vi "test_Compare Test Object Accessors.vi"() -> ()   [LabVIEW 2015]
uses:
  Test Object/Test Object.lvclass
  Test Object/Test Object.lvclass/Test Object.ctl
  Test Object/Read Variant (sta prop).vi
  Test Object/Write Variant (sta prop).vi
panel:
  out "Average test duration [ms]":dbl[][](array[numeric]) format="%#.6p"
  # "Access Variant w/o modification"
  # "Access and modify Variant in-place"
  # "Access and reallocate Variant"
  # "Static w/o errors"
  # "Dynam w/o errors"
  # "Static prop"
  # "Dynam prop"
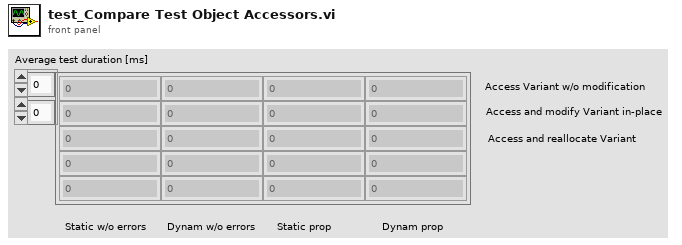
[diagram p1: front panel]
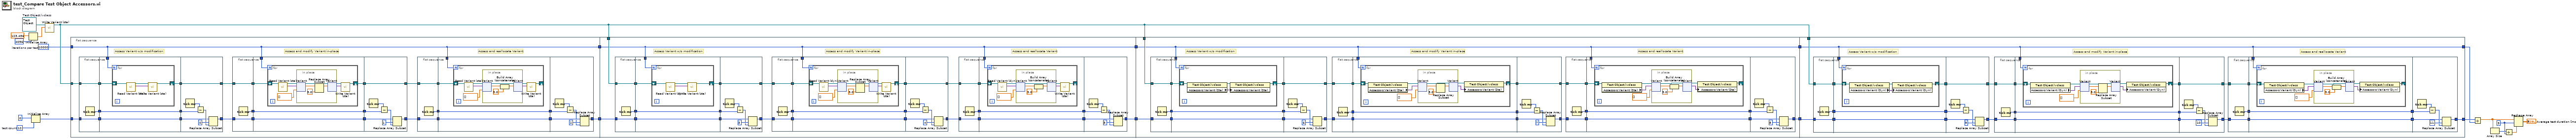
[diagram p0: block diagram]
diagram:
  w6 = 10000  # iterations per test
  w8 = 3
  w16 = 12  # test count
  w22 = refnum<class "Test Object.lvclass"> refnum  # Test Object.lvclass
  n1 = Initialize Array(123.456, 4096) -> (w19:dbl[])
  n2 = Initialize Array(u32 0, w16) -> (w15:u32[])
  n3 = call "Write Variant (sta).vi"("Variant"=w19, "Test Object in"=w22) -> ("Test Object out"=w18:refnum<class "Test Object.lvclass">)  [unwired: 9 in]
  n4 = flat-sequence {
    tunnel: w18 -> [w34]
    tunnel: w15 -> [w33]
    tunnel: [w24] -> w14
    tunnel: w6 -> [w23]
    tunnel: [w23] -> w5
    tunnel: w18 -> [w116]
    tunnel: w14 -> [w115]
    tunnel: [w114] -> w13
    tunnel: w5 -> [w113]
    tunnel: [w113] -> w4
    tunnel: w18 -> [w214]
    tunnel: w13 -> [w211]
    tunnel: [w204] -> w12
    tunnel: w4 -> [w203]
    tunnel: [w203] -> w3
    tunnel: w18 -> [w296]
    tunnel: w12 -> [w295]
    tunnel: [w294] -> w10
    tunnel: w3 -> [w293]
    tunnel: [w293] -> w1
    frame #0 {
      # "Access and reallocate Variant"
      # "Access and modify Variant in-place"
      # "Access Variant w/o modification"
      n5 = flat-sequence {
        tunnel: w34 -> [w96]
        tunnel: [w96] -> w47
        tunnel: [w95] -> w46
        tunnel: w33 -> [w94]
        tunnel: [w94] -> w32
        tunnel: w47 -> [w101]
        tunnel: w46 -> [w99]
        tunnel: [w100] -> w45
        tunnel: [w99] -> w44
        tunnel: w32 -> [w98]
        tunnel: [w98] -> w31
        tunnel: w23 -> [w97]
        tunnel: [w112] -> w35
        tunnel: w45 -> [w112]
        tunnel: w44 -> [w111]
        tunnel: w31 -> [w107]
        tunnel: [w106] -> w29
        frame #0 {
          n6 = Tick Count (ms)() -> (millisecond timer value=w95:u32)
        }
        frame #1 {
          n7 = for {
            N: w97 -> [_]
            shift-right: [w103] -> w100
            shift-left: w101 -> [w105]
            n8 = call "Read Variant (sta).vi"("Test Object in"=w105) -> ("Variant"=w102:variant, "Test Object out"=w104:refnum<class "Test Object.lvclass">)  [unwired: 9 in]
            n9 = call "Write Variant (sta).vi"("Variant"=w102, "Test Object in"=w104) -> ("Test Object out"=w103:refnum<class "Test Object.lvclass">)  [unwired: 9 in]
          }
        }
        frame #2 {
          n10 = Tick Count (ms)() -> (millisecond timer value=w110:u32)
          n11 = Subtract(x=w110, y=w111) -> (x-y=w108:u32)
          n12 = Replace Array Subset(array=w107, new element=w108, index=0) -> (w106:u32[])
        }
      }
      n13 = flat-sequence {
        tunnel: w35 -> [w72]
        tunnel: [w72] -> w43
        tunnel: [w71] -> w42
        tunnel: [w70] -> w30
        tunnel: w29 -> [w70]
        tunnel: w43 -> [w77]
        tunnel: w42 -> [w75]
        tunnel: [w76] -> w41
        tunnel: [w75] -> w40
        tunnel: w30 -> [w74]
        tunnel: [w74] -> w28
        tunnel: w23 -> [w73]
        tunnel: [w93] -> w36
        tunnel: w41 -> [w93]
        tunnel: w40 -> [w92]
        tunnel: w28 -> [w88]
        tunnel: [w87] -> w26
        frame #0 {
          n14 = Tick Count (ms)() -> (millisecond timer value=w71:u32)
        }
        frame #1 {
          n15 = for {
            N: w73 -> [_]
            shift-right: [w81] -> w76
            shift-left: w77 -> [w83]
            n16 = call "Read Variant (sta).vi"("Test Object in"=w83) -> ("Variant"=w80:variant, "Test Object out"=w82:refnum<class "Test Object.lvclass">)  [unwired: 9 in]
            n17 = in-place {
              n18 = in-place-variant #1(w80, dbl[] []) -> (w86:dbl[])  [unwired: 1 out]
              n19 = Replace Array Subset(array=w86, new element=5.0) -> (w85:dbl[])  [unwired: 1 in]
              n20 = in-place-variant #1(w85) -> (w79:variant)  [unwired: 1 out]
            }
            n21 = call "Write Variant (sta).vi"("Variant"=w79, "Test Object in"=w82) -> ("Test Object out"=w81:refnum<class "Test Object.lvclass">)  [unwired: 9 in]
          }
        }
        frame #2 {
          n22 = Tick Count (ms)() -> (millisecond timer value=w91:u32)
          n23 = Subtract(x=w91, y=w92) -> (x-y=w89:u32)
          n24 = Replace Array Subset(array=w88, new element=w89, index=1) -> (w87:u32[])
        }
      }
      n25 = flat-sequence {
        tunnel: w36 -> [w50]
        tunnel: [w50] -> w39
        tunnel: [w49] -> w38
        tunnel: [w48] -> w27
        tunnel: w26 -> [w48]
        tunnel: w39 -> [w54]
        tunnel: w38 -> [w53]
        tunnel: [w53] -> w37
        tunnel: w27 -> [w52]
        tunnel: [w52] -> w25
        tunnel: w23 -> [w51]
        tunnel: w37 -> [w69]
        tunnel: w25 -> [w66]
        tunnel: [w64] -> w24
        frame #0 {
          n26 = Tick Count (ms)() -> (millisecond timer value=w49:u32)
        }
        frame #1 {
          n27 = for {
            N: w51 -> [_]
            shift-right: [w58] -> _
            shift-left: w54 -> [w60]
            n28 = call "Read Variant (sta).vi"("Test Object in"=w60) -> ("Variant"=w57:variant, "Test Object out"=w59:refnum<class "Test Object.lvclass">)  [unwired: 9 in]
            n29 = in-place {
              n30 = in-place-variant #2(w57, dbl[] []) -> (w63:dbl[])  [unwired: 1 out]
              n31 = Build Array (concatenate)(w63, 5.0) -> (w62:dbl[])
              n32 = in-place-variant #2(w62) -> (w56:variant)  [unwired: 1 out]
            }
            n33 = call "Write Variant (sta).vi"("Variant"=w56, "Test Object in"=w59) -> ("Test Object out"=w58:refnum<class "Test Object.lvclass">)  [unwired: 9 in]
          }
        }
        frame #2 {
          n34 = Tick Count (ms)() -> (millisecond timer value=w68:u32)
          n35 = Subtract(x=w68, y=w69) -> (x-y=w65:u32)
          n36 = Replace Array Subset(array=w66, new element=w65, index=2) -> (w64:u32[])
        }
      }
    }
    frame #1 {
      # "Access and reallocate Variant"
      # "Access and modify Variant in-place"
      # "Access Variant w/o modification"
      n37 = flat-sequence {
        tunnel: w116 -> [w186]
        tunnel: [w186] -> w137
        tunnel: [w185] -> w136
        tunnel: w115 -> [w184]
        tunnel: [w184] -> w135
        tunnel: w137 -> [w191]
        tunnel: w136 -> [w189]
        tunnel: [w190] -> w134
        tunnel: [w189] -> w133
        tunnel: w135 -> [w188]
        tunnel: [w188] -> w132
        tunnel: w113 -> [w187]
        tunnel: [w202] -> w119
        tunnel: w134 -> [w202]
        tunnel: w133 -> [w201]
        tunnel: w132 -> [w197]
        tunnel: [w196] -> w118
        frame #0 {
          n38 = Tick Count (ms)() -> (millisecond timer value=w185:u32)
        }
        frame #1 {
          n39 = for {
            N: w187 -> [_]
            shift-right: [w193] -> w190
            shift-left: w191 -> [w195]
            n40 = call-dynamic "Read Variant (dyn).vi"("Test Object in"=w195) -> ("Variant"=w192:variant, "Test Object out"=w194:refnum<class "Test Object.lvclass">)  [unwired: 9 in]
            n41 = call "Write Variant (sta).vi"("Variant"=w192, "Test Object in"=w194) -> ("Test Object out"=w193:refnum<class "Test Object.lvclass">)  [unwired: 9 in]
          }
        }
        frame #2 {
          n42 = Tick Count (ms)() -> (millisecond timer value=w200:u32)
          n43 = Subtract(x=w200, y=w201) -> (x-y=w198:u32)
          n44 = Replace Array Subset(array=w197, new element=w198, index=3) -> (w196:u32[])
        }
      }
      n45 = flat-sequence {
        tunnel: w119 -> [w162]
        tunnel: [w162] -> w131
        tunnel: [w161] -> w130
        tunnel: [w160] -> w129
        tunnel: w118 -> [w160]
        tunnel: w131 -> [w167]
        tunnel: w130 -> [w165]
        tunnel: [w166] -> w128
        tunnel: [w165] -> w127
        tunnel: w129 -> [w164]
        tunnel: [w164] -> w126
        tunnel: w113 -> [w163]
        tunnel: [w183] -> w120
        tunnel: w128 -> [w183]
        tunnel: w127 -> [w182]
        tunnel: w126 -> [w178]
        tunnel: [w177] -> w117
        frame #0 {
          n46 = Tick Count (ms)() -> (millisecond timer value=w161:u32)
        }
        frame #1 {
          n47 = for {
            N: w163 -> [_]
            shift-right: [w171] -> w166
            shift-left: w167 -> [w173]
            n48 = call-dynamic "Read Variant (dyn).vi"("Test Object in"=w173) -> ("Variant"=w170:variant, "Test Object out"=w172:refnum<class "Test Object.lvclass">)  [unwired: 9 in]
            n49 = in-place {
              n50 = in-place-variant #3(w170, dbl[] []) -> (w176:dbl[])  [unwired: 1 out]
              n51 = Replace Array Subset(array=w176, new element=5.0) -> (w175:dbl[])  [unwired: 1 in]
              n52 = in-place-variant #3(w175) -> (w169:variant)  [unwired: 1 out]
            }
            n53 = call "Write Variant (sta).vi"("Variant"=w169, "Test Object in"=w172) -> ("Test Object out"=w171:refnum<class "Test Object.lvclass">)  [unwired: 9 in]
          }
        }
        frame #2 {
          n54 = Tick Count (ms)() -> (millisecond timer value=w181:u32)
          n55 = Subtract(x=w181, y=w182) -> (x-y=w179:u32)
          n56 = Replace Array Subset(array=w178, new element=w179, index=4) -> (w177:u32[])
        }
      }
      n57 = flat-sequence {
        tunnel: w120 -> [w140]
        tunnel: [w140] -> w125
        tunnel: [w139] -> w124
        tunnel: [w138] -> w123
        tunnel: w117 -> [w138]
        tunnel: w125 -> [w144]
        tunnel: w124 -> [w143]
        tunnel: [w143] -> w122
        tunnel: w123 -> [w142]
        tunnel: [w142] -> w121
        tunnel: w113 -> [w141]
        tunnel: w122 -> [w159]
        tunnel: w121 -> [w156]
        tunnel: [w154] -> w114
        frame #0 {
          n58 = Tick Count (ms)() -> (millisecond timer value=w139:u32)
        }
        frame #1 {
          n59 = for {
            N: w141 -> [_]
            shift-right: [w148] -> _
            shift-left: w144 -> [w150]
            n60 = call-dynamic "Read Variant (dyn).vi"("Test Object in"=w150) -> ("Variant"=w147:variant, "Test Object out"=w149:refnum<class "Test Object.lvclass">)  [unwired: 9 in]
            n61 = in-place {
              n62 = in-place-variant #4(w147, dbl[] []) -> (w153:dbl[])  [unwired: 1 out]
              n63 = Build Array (concatenate)(w153, 5.0) -> (w152:dbl[])
              n64 = in-place-variant #4(w152) -> (w146:variant)  [unwired: 1 out]
            }
            n65 = call "Write Variant (sta).vi"("Variant"=w146, "Test Object in"=w149) -> ("Test Object out"=w148:refnum<class "Test Object.lvclass">)  [unwired: 9 in]
          }
        }
        frame #2 {
          n66 = Tick Count (ms)() -> (millisecond timer value=w158:u32)
          n67 = Subtract(x=w158, y=w159) -> (x-y=w155:u32)
          n68 = Replace Array Subset(array=w156, new element=w155, index=5) -> (w154:u32[])
        }
      }
    }
    frame #2 {
      # "Access and reallocate Variant"
      # "Access and modify Variant in-place"
      # "Access Variant w/o modification"
      n69 = flat-sequence {
        tunnel: w214 -> [w276]
        tunnel: [w276] -> w227
        tunnel: [w275] -> w226
        tunnel: [w274] -> w212
        tunnel: w211 -> [w274]
        tunnel: w227 -> [w281]
        tunnel: w226 -> [w279]
        tunnel: [w280] -> w225
        tunnel: [w279] -> w224
        tunnel: [w278] -> w213
        tunnel: w212 -> [w278]
        tunnel: w203 -> [w277]
        tunnel: [w292] -> w216
        tunnel: w225 -> [w292]
        tunnel: w224 -> [w291]
        tunnel: w213 -> [w288]
        tunnel: [w286] -> w208
        frame #0 {
          n70 = Tick Count (ms)() -> (millisecond timer value=w275:u32)
        }
        frame #1 {
          n71 = for {
            N: w277 -> [_]
            shift-right: [w283] -> w280
            shift-left: w281 -> [w285]
            n72 = property class="Test Object.lvclass"(reference=w285) -> (reference out=w284:refnum<class "Test Object.lvclass">, "Accessors:Variant (Sta)"=w282:variant)  [unwired: 1 in, 1 out]
            n73 = property class="Test Object.lvclass"(reference=w284, "Accessors:Variant (Sta)"=w282) -> (reference out=w283:refnum<class "Test Object.lvclass">)  [unwired: 1 in, 1 out]
          }
        }
        frame #2 {
          n74 = Tick Count (ms)() -> (millisecond timer value=w290:u32)
          n75 = Subtract(x=w290, y=w291) -> (x-y=w287:u32)
          n76 = Replace Array Subset(array=w288, new element=w287, index=6) -> (w286:u32[])
        }
      }
      n77 = flat-sequence {
        tunnel: w216 -> [w252]
        tunnel: [w252] -> w223
        tunnel: [w251] -> w222
        tunnel: [w250] -> w209
        tunnel: w208 -> [w250]
        tunnel: w223 -> [w257]
        tunnel: w222 -> [w255]
        tunnel: [w256] -> w221
        tunnel: [w255] -> w220
        tunnel: [w254] -> w210
        tunnel: w209 -> [w254]
        tunnel: w203 -> [w253]
        tunnel: [w273] -> w215
        tunnel: w221 -> [w273]
        tunnel: w220 -> [w272]
        tunnel: w210 -> [w268]
        tunnel: [w267] -> w206
        frame #0 {
          n78 = Tick Count (ms)() -> (millisecond timer value=w251:u32)
        }
        frame #1 {
          n79 = for {
            N: w253 -> [_]
            shift-right: [w261] -> w256
            shift-left: w257 -> [w263]
            n80 = property class="Test Object.lvclass"(reference=w263) -> (reference out=w262:refnum<class "Test Object.lvclass">, "Accessors:Variant (Sta)"=w259:variant)  [unwired: 1 in, 1 out]
            n81 = in-place {
              n82 = in-place-variant #5(w259, dbl[] []) -> (w266:dbl[])  [unwired: 1 out]
              n83 = Replace Array Subset(array=w266, new element=5.0) -> (w265:dbl[])  [unwired: 1 in]
              n84 = in-place-variant #5(w265) -> (w258:variant)  [unwired: 1 out]
            }
            n85 = property class="Test Object.lvclass"(reference=w262, "Accessors:Variant (Sta)"=w258) -> (reference out=w261:refnum<class "Test Object.lvclass">)  [unwired: 1 in, 1 out]
          }
        }
        frame #2 {
          n86 = Tick Count (ms)() -> (millisecond timer value=w271:u32)
          n87 = Subtract(x=w271, y=w272) -> (x-y=w269:u32)
          n88 = Replace Array Subset(array=w268, new element=w269, index=7) -> (w267:u32[])
        }
      }
      n89 = flat-sequence {
        tunnel: w215 -> [w230]
        tunnel: [w230] -> w219
        tunnel: [w229] -> w218
        tunnel: [w228] -> w207
        tunnel: w206 -> [w228]
        tunnel: w219 -> [w234]
        tunnel: w218 -> [w233]
        tunnel: [w233] -> w217
        tunnel: w207 -> [w232]
        tunnel: [w232] -> w205
        tunnel: w203 -> [w231]
        tunnel: w217 -> [w249]
        tunnel: w205 -> [w245]
        tunnel: [w244] -> w204
        frame #0 {
          n90 = Tick Count (ms)() -> (millisecond timer value=w229:u32)
        }
        frame #1 {
          n91 = for {
            N: w231 -> [_]
            shift-right: [w238] -> _
            shift-left: w234 -> [w240]
            n92 = property class="Test Object.lvclass"(reference=w240) -> (reference out=w239:refnum<class "Test Object.lvclass">, "Accessors:Variant (Sta)"=w236:variant)  [unwired: 1 in, 1 out]
            n93 = in-place {
              n94 = in-place-variant #6(w236, dbl[] []) -> (w243:dbl[])  [unwired: 1 out]
              n95 = Build Array (concatenate)(w243, 5.0) -> (w242:dbl[])
              n96 = in-place-variant #6(w242) -> (w235:variant)  [unwired: 1 out]
            }
            n97 = property class="Test Object.lvclass"(reference=w239, "Accessors:Variant (Sta)"=w235) -> (reference out=w238:refnum<class "Test Object.lvclass">)  [unwired: 1 in, 1 out]
          }
        }
        frame #2 {
          n98 = Tick Count (ms)() -> (millisecond timer value=w248:u32)
          n99 = Subtract(x=w248, y=w249) -> (x-y=w246:u32)
          n100 = Replace Array Subset(array=w245, new element=w246, index=8) -> (w244:u32[])
        }
      }
    }
    frame #3 {
      # "Access and reallocate Variant"
      # "Access and modify Variant in-place"
      # "Access Variant w/o modification"
      n101 = flat-sequence {
        tunnel: w296 -> [w366]
        tunnel: [w366] -> w317
        tunnel: [w365] -> w316
        tunnel: [w364] -> w315
        tunnel: w295 -> [w364]
        tunnel: w317 -> [w371]
        tunnel: w316 -> [w369]
        tunnel: [w370] -> w314
        tunnel: [w369] -> w313
        tunnel: [w368] -> w312
        tunnel: w315 -> [w368]
        tunnel: w293 -> [w367]
        tunnel: [w382] -> w300
        tunnel: w314 -> [w382]
        tunnel: w313 -> [w381]
        tunnel: w312 -> [w378]
        tunnel: [w376] -> w298
        frame #0 {
          n102 = Tick Count (ms)() -> (millisecond timer value=w365:u32)
        }
        frame #1 {
          n103 = for {
            N: w367 -> [_]
            shift-right: [w373] -> w370
            shift-left: w371 -> [w375]
            n104 = property class="Test Object.lvclass"(reference=w375) -> (reference out=w374:refnum<class "Test Object.lvclass">, "Accessors:Variant (Dyn)"=w372:variant)  [unwired: 1 in, 1 out]
            n105 = property class="Test Object.lvclass"(reference=w374, "Accessors:Variant (Dyn)"=w372) -> (reference out=w373:refnum<class "Test Object.lvclass">)  [unwired: 1 in, 1 out]
          }
        }
        frame #2 {
          n106 = Tick Count (ms)() -> (millisecond timer value=w380:u32)
          n107 = Subtract(x=w380, y=w381) -> (x-y=w377:u32)
          n108 = Replace Array Subset(array=w378, new element=w377, index=9) -> (w376:u32[])
        }
      }
      n109 = flat-sequence {
        tunnel: w300 -> [w342]
        tunnel: [w342] -> w311
        tunnel: [w341] -> w310
        tunnel: [w340] -> w309
        tunnel: w298 -> [w340]
        tunnel: w311 -> [w347]
        tunnel: w310 -> [w345]
        tunnel: [w346] -> w308
        tunnel: [w345] -> w307
        tunnel: [w344] -> w306
        tunnel: w309 -> [w344]
        tunnel: w293 -> [w343]
        tunnel: [w363] -> w299
        tunnel: w308 -> [w363]
        tunnel: w307 -> [w362]
        tunnel: w306 -> [w358]
        tunnel: [w357] -> w297
        frame #0 {
          n110 = Tick Count (ms)() -> (millisecond timer value=w341:u32)
        }
        frame #1 {
          n111 = for {
            N: w343 -> [_]
            shift-right: [w351] -> w346
            shift-left: w347 -> [w353]
            n112 = property class="Test Object.lvclass"(reference=w353) -> (reference out=w352:refnum<class "Test Object.lvclass">, "Accessors:Variant (Dyn)"=w349:variant)  [unwired: 1 in, 1 out]
            n113 = in-place {
              n114 = in-place-variant #7(w349, dbl[] []) -> (w356:dbl[])  [unwired: 1 out]
              n115 = Replace Array Subset(array=w356, new element=5.0) -> (w355:dbl[])  [unwired: 1 in]
              n116 = in-place-variant #7(w355) -> (w348:variant)  [unwired: 1 out]
            }
            n117 = property class="Test Object.lvclass"(reference=w352, "Accessors:Variant (Dyn)"=w348) -> (reference out=w351:refnum<class "Test Object.lvclass">)  [unwired: 1 in, 1 out]
          }
        }
        frame #2 {
          n118 = Tick Count (ms)() -> (millisecond timer value=w361:u32)
          n119 = Subtract(x=w361, y=w362) -> (x-y=w359:u32)
          n120 = Replace Array Subset(array=w358, new element=w359, index=10) -> (w357:u32[])
        }
      }
      n121 = flat-sequence {
        tunnel: w299 -> [w320]
        tunnel: [w320] -> w305
        tunnel: [w319] -> w304
        tunnel: [w318] -> w303
        tunnel: w297 -> [w318]
        tunnel: w305 -> [w324]
        tunnel: w304 -> [w323]
        tunnel: [w323] -> w302
        tunnel: w303 -> [w322]
        tunnel: [w322] -> w301
        tunnel: w293 -> [w321]
        tunnel: w302 -> [w339]
        tunnel: w301 -> [w335]
        tunnel: [w334] -> w294
        frame #0 {
          n122 = Tick Count (ms)() -> (millisecond timer value=w319:u32)
        }
        frame #1 {
          n123 = for {
            N: w321 -> [_]
            shift-right: [w328] -> _
            shift-left: w324 -> [w330]
            n124 = property class="Test Object.lvclass"(reference=w330) -> (reference out=w329:refnum<class "Test Object.lvclass">, "Accessors:Variant (Dyn)"=w326:variant)  [unwired: 1 in, 1 out]
            n125 = in-place {
              n126 = in-place-variant #8(w326, dbl[] []) -> (w333:dbl[])  [unwired: 1 out]
              n127 = Build Array (concatenate)(w333, 5.0) -> (w332:dbl[])
              n128 = in-place-variant #8(w332) -> (w325:variant)  [unwired: 1 out]
            }
            n129 = property class="Test Object.lvclass"(reference=w329, "Accessors:Variant (Dyn)"=w325) -> (reference out=w328:refnum<class "Test Object.lvclass">)  [unwired: 1 in, 1 out]
          }
        }
        frame #2 {
          n130 = Tick Count (ms)() -> (millisecond timer value=w338:u32)
          n131 = Subtract(x=w338, y=w339) -> (x-y=w336:u32)
          n132 = Replace Array Subset(array=w335, new element=w336, index=11) -> (w334:u32[])
        }
      }
    }
  }
  n133 = Divide(x=w10, y=w1) -> (x/y=w2:dbl[])
  n134 = Array Size(array=w2) -> (size(s)=w9:i32)
  n135 = Divide(x=w9, y=w8) -> (x/y=w7:dbl)
  n136 = Reshape Array(w2, w8, w7) -> (→"Average test duration [ms]":dbl[][])
